vi "Finalize Settings 1.0.vi"(8 "error in (no error)":errorcluster, 11 "configuration 1.0":T2={"name"="Channel", "units"="V", "engine data type"=enum."DBL", "string data type"=enum."DBL", "string offset"=0} {"string offset" format="%d bytes"}) -> (0 "error out":errorcluster, 2 "settings version":T1, 3 "settings 1.0":cluster{"key":string, "value":string}[](array[cluster]))   [LabVIEW 2021, in "DSF Core.lvlib" / "Channel Configuration.lvclass"]
uses:
  Channel Configuration.lvclass
  Typedefs/DSF Version Info.ctl
  DSF Core.lvlib
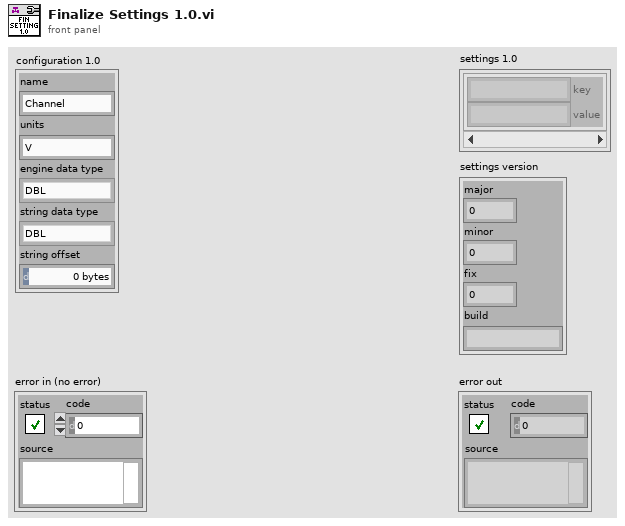
[diagram p1: front panel]
types:
  T1 = typedef "DSF Core.lvlib/DSF Version Info.ctl" = cluster{"major":u32, "minor":u32, "fix":u32, "build":string}
  T2 = cluster{"name":string, "units":string, "engine data type":enum8{"Bool", "SGL", "DBL", "I8", "I16", "I32", "I64", "U8", "U16", "U32", "U64"}, "string data type":enum8{"Bool", "SGL", "DBL", "I8", "I16", "I32", "I64", "U8", "U16", "U32", "U64"}, "string offset":u64}
  T3 = enum8{"Bool", "SGL", "DBL", "I8", "I16", "I32", "I64", "U8", "U16", "U32", "U64"}
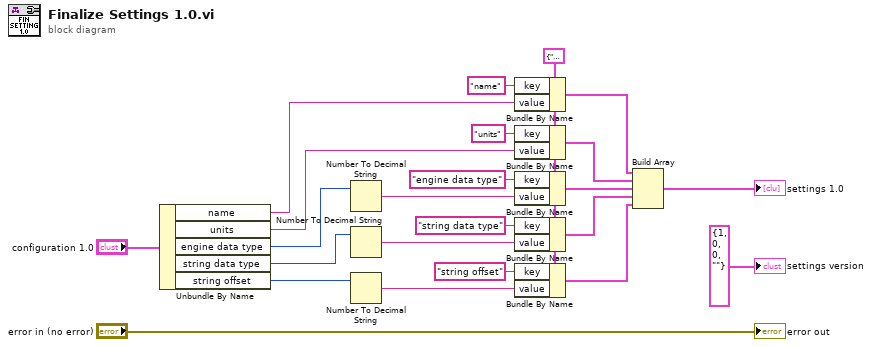
[diagram p0: block diagram]
diagram:
  w4 = cluster{"key":string, "value":string} {"key"="", "value"=""} ("setting")
  n1 = Unbundle By Name("configuration 1.0") -> ("name"=w14:string, "units"=w13:string, "engine data type"=w9:T3, "string data type"=w8:T3, "string offset"=w7:u64)
  n2 = Number To Decimal String(number=w9) -> (decimal integer string=w12:string)  [unwired: 1 in]
  n3 = Number To Decimal String(number=w8) -> (decimal integer string=w11:string)  [unwired: 1 in]
  n4 = Number To Decimal String(number=w7) -> (decimal integer string=w10:string)  [unwired: 1 in]
  n5 = Bundle By Name(cluster=w4, "key"="name", "value"=w14) -> (w23:cluster{"key":string, "value":string})
  n6 = Bundle By Name(cluster=w4, "key"="units", "value"=w13) -> (w22:cluster{"key":string, "value":string})
  n7 = Bundle By Name(cluster=w4, "key"="engine data type", "value"=w12) -> (w21:cluster{"key":string, "value":string})
  n8 = Bundle By Name(cluster=w4, "key"="string data type", "value"=w11) -> (w20:cluster{"key":string, "value":string})
  n9 = Bundle By Name(cluster=w4, "key"="string offset", "value"=w10) -> (w3:cluster{"key":string, "value":string})
  n10 = Build Array(w23, w22, w21, w20, w3) -> (→"settings 1.0":cluster{"key":string, "value":string}[])
  "error out" <- "error in (no error)"
  "settings version" <- T1 {"major"=1, "minor"=0, "fix"=0, "build"=""} ("settings version")
